vi "pcfs_abort_dither.vi"(8 "error in (no error)":errorcluster, 11 "pcfs in":refnum<class "pcfs.lvclass">) -> (0 "error out":errorcluster, 3 "pcfs out":refnum<class "pcfs.lvclass">)   [LabVIEW 2015, in "pcfs.lvclass"]
uses:
  pcfs.lvclass
  pcfs.lvclass/pcfs.ctl
  Stage Class/Stage.lvclass
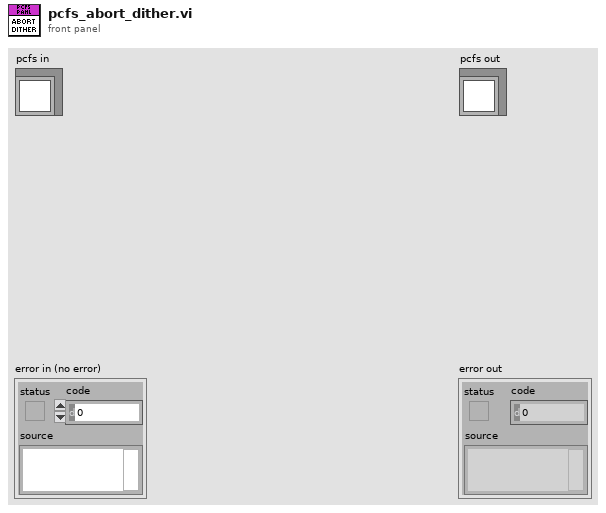
[diagram p1: front panel]
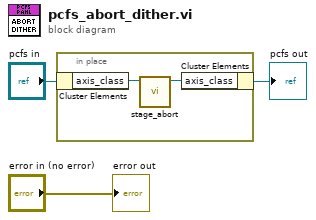
[diagram p0: block diagram]
diagram:
  n1 = in-place {
    n2 = in-place-cluster #1("pcfs in") -> ("axis_class"=w5:refnum<class "Stage.lvclass">)
    n3 = call-dynamic "stage_abort.vi"("Stage in"=w5) -> ("Stage out"=w4:refnum<class "Stage.lvclass">)  [unwired: 9 in, 1 out]
    n4 = in-place-cluster #1("axis_class"=w4) -> (→"pcfs out":refnum<class "pcfs.lvclass">)
  }
  "error out" <- "error in (no error)"
